vi "EMB_Debug_Map_RV_UpdateDD.vi"(6 "RDM":bool=TRUE, 8 "error in (no error)":errorcluster, 10 "Build Path":path, 11 "Source Path":path) -> (0 "error out":errorcluster, 3 "VI Name":string)   [LabVIEW 2011]
uses:
  <vilib>/LabVIEW Targets/Embedded/Debug/DD/utils/EMB_Debug_DD_Error.ctl
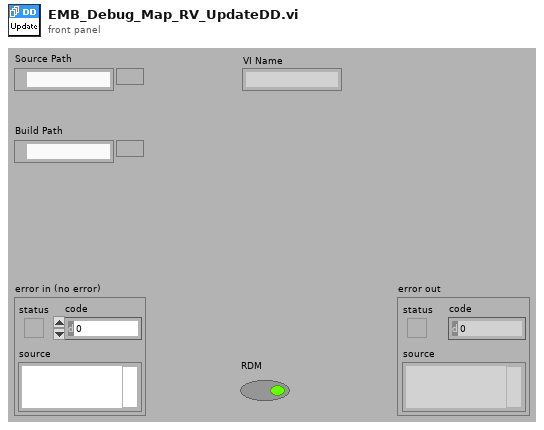
[diagram p1: front panel]
types:
  T1 = typedef "EMB_Debug_DD_Error.ctl" = enum16{"NoErr", "ErrNotFound", "ErrMemAlloc", "ErrLineNumberKeyViolation", "ErrAddressKeyViolation", "ErrIndexKeyViolation", "ErrSignalKeyViolation", "ErrControlKeyViolation", "ErrStructItemKeyViolation", "ErrInvalidTargetID", "ErrSyntaxError", "ErrParseVIName", "ErrParseCFile", "ErrSymbolNotFound", "ErrImplNotFound", "ErrDuplicateNodeEnd", "ErrOrphanNodeEnd"}
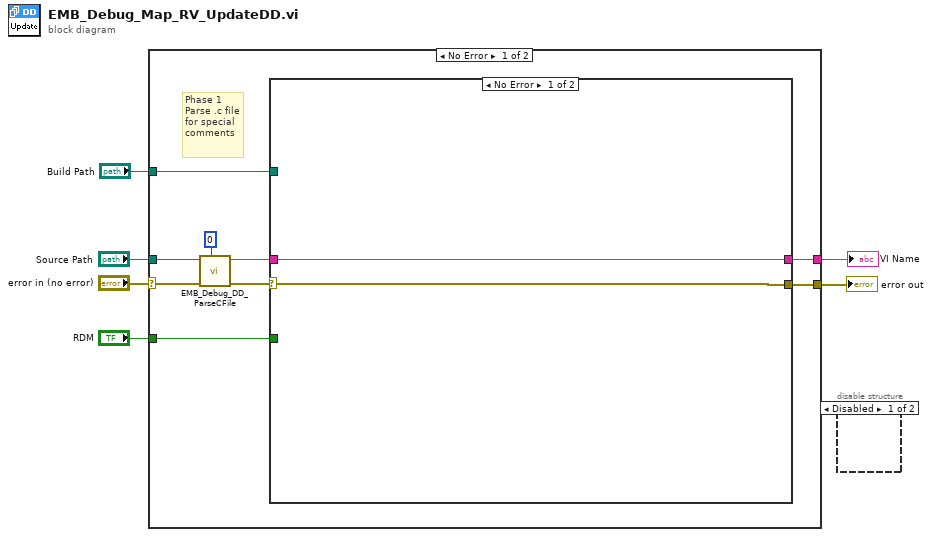
[diagram p0: block diagram]
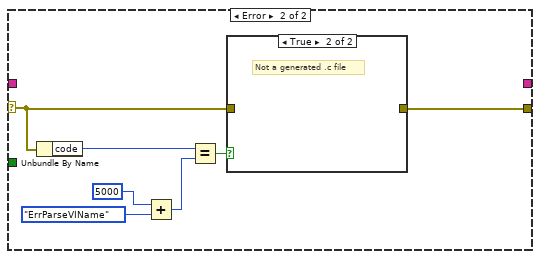
[diagram p3: hidden frame]
diagram:
  n1 = case shown="No Error" "error in (no error)" {
    selector: "error in (no error)" -> [w15 w26]
    tunnel: "Source Path" -> [w14 _]
    tunnel: [w11 w26] -> w4
    tunnel: "Build Path" -> [w10 _]
    tunnel: "RDM" -> [w9 _]
    tunnel: [w7 _] -> w1
    frame No Error {
      # "Phase 1\nParse .c file for special comments"
      n2 = call <vilib>:"EMB_Debug_DD_ParseCFile.vi"("target ID"=u32 0, "error in (no error)"=w15, "Path"=w14) -> ("error out"=w13:errorcluster, "VI Name"=w12:string)  [unwired: 7 in]
      n3 = case shown="No Error" w13 {
        selector: w13 -> [w17 w19]
        tunnel: w12 -> [w16 _]
        tunnel: [w17 w18] -> w11
        tunnel: w10 -> [_ _]
        tunnel: w9 -> [_ _]
        tunnel: [w16 _] -> w7
        frame No Error {
        }
        frame Error {
          n4 = Unbundle By Name(w19) -> ("code"=w22:i32)
          n5 = Add(x=5000, y=EMB_Debug_DD_Error."ErrParseVIName" ("Error")) -> (x+y=w21:i32)
          n6 = Equal?(x=w22, y=w21) -> (x = y?=w20:bool)
          n7 = case shown="True" w20 {
            tunnel: w19 -> [w25 _]
            tunnel: [w25 _] -> w18
            frame False {
            }
            frame True {
              # "Not a generated .c file"
            }
          }
        }
      }
    }
    frame Error {
    }
  }
  "error out" <- w4
  "VI Name" <- w1
  n8 = disable-structure shown="Disabled" {
    frame Disabled {
    }
    frame Enabled {
    }
  }
